vi "CPU_RESET_handle.vi"(11 "registers":T1 {"P" format="%08b"; "PC" format="%04x"; "SP" format="%02x"; "Y" format="%02x"; "X" format="%02x"; "A" format="%02x"}) -> (3 "registers":T1 {"P" format="%08b"; "PC" format="%04x"; "SP" format="%02x"; "Y" format="%02x"; "X" format="%02x"; "A" format="%02x"})   [LabVIEW 2018]
uses:
  CPU_registers.ctl
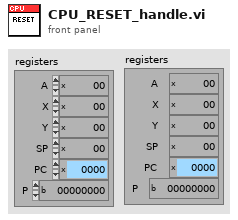
[diagram p1: front panel]
types:
  T1 = typedef "CPU_registers.ctl" = cluster{"A":u8, "X":u8, "Y":u8, "SP":u8, "PC":u16, "P":u8}
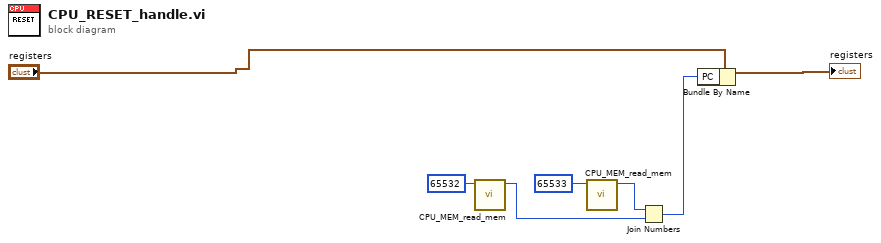
[diagram p0: block diagram]
diagram:
  n1 = call "CPU_MEM_read_mem.vi"("address"=u16 65532) -> ("value out"=w5:u8)  [unwired: 10 in]
  n2 = call "CPU_MEM_read_mem.vi"("address"=u16 65533) -> ("value out"=w4:u8)  [unwired: 10 in]
  n3 = Join Numbers(hi=w4, lo=w5) -> ((hi.lo)=w1:u16)
  n4 = Bundle By Name(cluster="registers", "PC"=w1) -> (→"registers":T1)
